vi "Set Upper Threshold Level [UPL].vi"(7 "Micropulse # In":i32, 8 "error in (no error)":errorcluster, 9 "Threshold":u16, 11 "Test Number":u32) -> (0 "error out":errorcluster, 5 "Micropulse # Out":i32)   [LabVIEW 2026, in "MicroPulse_Driver.lvlib"]
doc: "Specifies the UPPER reporting threshold for the specified Test Number (Tn). Any signals ABOVE the UPL threshold level value and within the search gate area will be recognised by the signal processor as possible valid peaks, depending on HYS. If no EUPL is specified, then the UPL is used in the interface gate in echo gate mode.\n\nParameters:\n<Tn> : Test number. An integer value from 0 to the maximum number of tests (default maximum is 1279 tests).\nTn = 0 for all conventional tests. If the S extension is used it applies to all tests in the sweep number specified: 1-32, 0 = all sweeps\n\n<Value> : Integer between 10 and 255 ( 8-bit modes)\nInteger between 10 and 1023 (10-bit modes)\nInteger between 10 and 4095 (12-bit modes)\n\nExample:\nUPL 6 80 : Assign a reporting threshold of 80 machine units to Test Number 6."
uses:
  MicroPulse_Driver.lvlib
  Private/MP-Registry Action-Enum.ctl
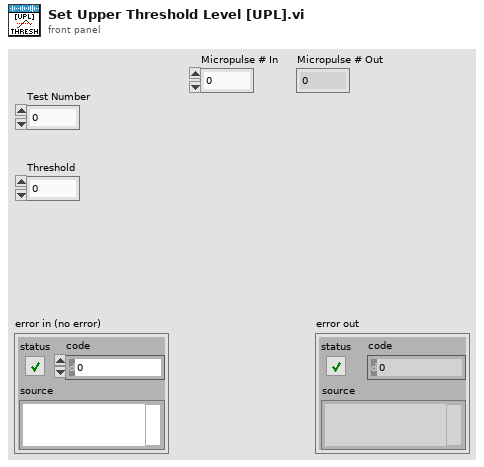
[diagram p1: front panel]
types:
  T1 = typedef "MicroPulse_Driver.lvlib/MP-Registry Action-Enum.ctl" = enum16{"Read", "Add Test", "Add Command", "Add Gate Command", "Add Encoder Command", "Clear Command  List", "Set Registry", "Set System Details", "Set DOF", "Set Velocity", "Disable Asynch Reads", "Enable Asynch Reads", "Add Connection", "Disconnect", "Shutdown"}
  T2 = typedef "Micropulse.lvlib/TCP config.ctl" = cluster{"Connection ID":refnum<k5>, "IP address":string, "host port":u16, "OC timeout":i32, "Read timeout":i32, "Write timeout":i32}
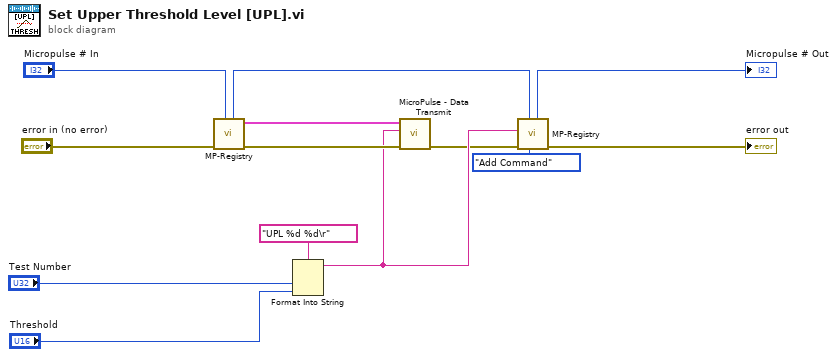
[diagram p0: block diagram]
diagram:
  n1 = call "MP-Registry.vi"("Micropulse # In"="Micropulse # In", "error in (no error)"="error in (no error)") -> ("error out"=w11:errorcluster, "TCP config"=w10:T2, "Micropulse # Out"=w4:i32)  [unwired: 6 in, 1 out]
  n2 = Format Into String(format string="UPL %d %d\r", "Test Number", "Threshold") -> (resulting string=w8:string)  [unwired: 2 in, 1 out]
  n3 = call "MicroPulse - Data Transmit.vi"("error in (no error)"=w11, "data"=w8, "TCP config"=w10) -> ("error out"=w6:errorcluster)  [unwired: 6 in, 2 out]
  n4 = call "MP-Registry.vi"("Action"=MP-Registry_Action-Enum."Add Command", "Micropulse # In"=w4, "error in (no error)"=w6, "Data in"=w8) -> ("error out"=→"error out":errorcluster, "Micropulse # Out"=→"Micropulse # Out":i32)  [unwired: 4 in, 2 out]
